vi "test_char limit case 1.vi"(8 "error in (no error)":errorcluster, 11 "TestCase in":refnum<class "Char Count Limit.lvclass">) -> (0 "error out":errorcluster, 3 "TestCase out":refnum<class "Char Count Limit.lvclass">)   [LabVIEW 2017, in "Char Count Limit.lvclass"]
uses:
  Char Count Limit.lvclass
  <vilib>/addons/_JKI Toolkits/VI Tester/TestCase.llb/TestCase.lvclass
  Libraries/SSH/SSH.lvlib
  C:/Program Files (x86)/National Instruments/LabVIEW 2017/vi.lib/addons/_JKI Toolkits/VI Tester/TestCase.llb/TestCase.lvclass
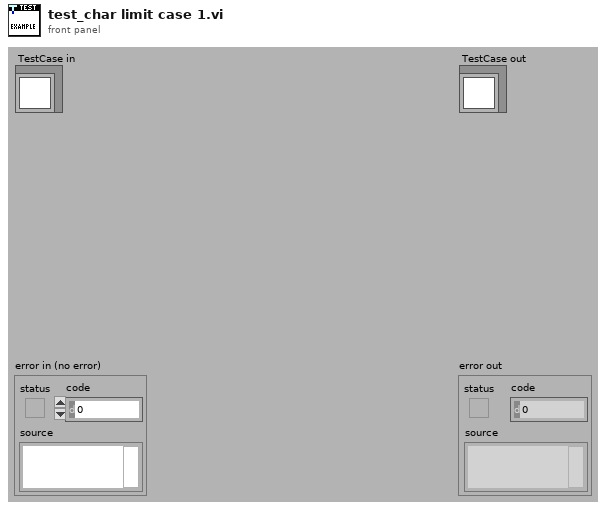
[diagram p1: front panel]
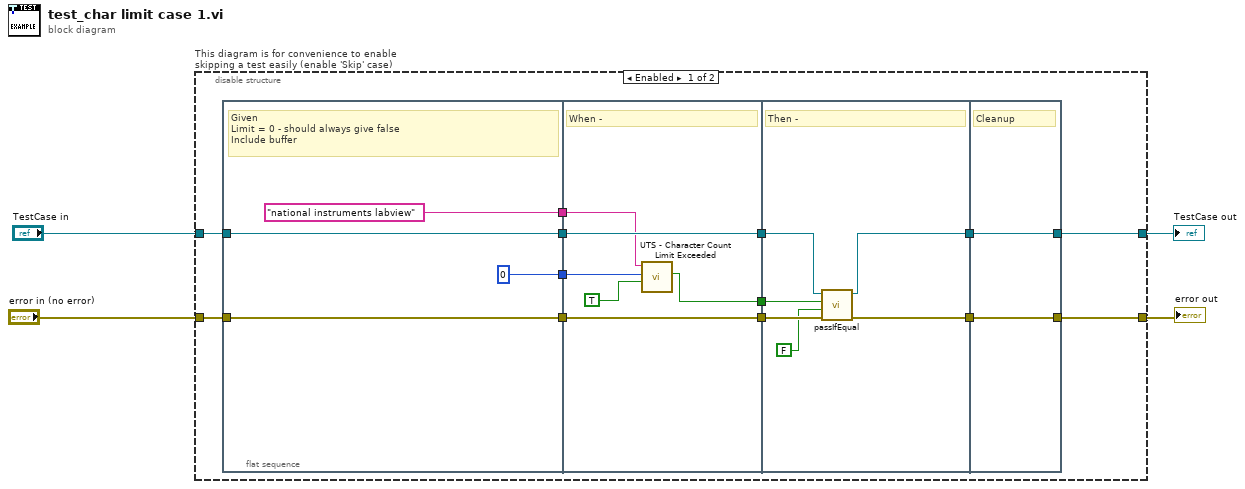
[diagram p0: block diagram]
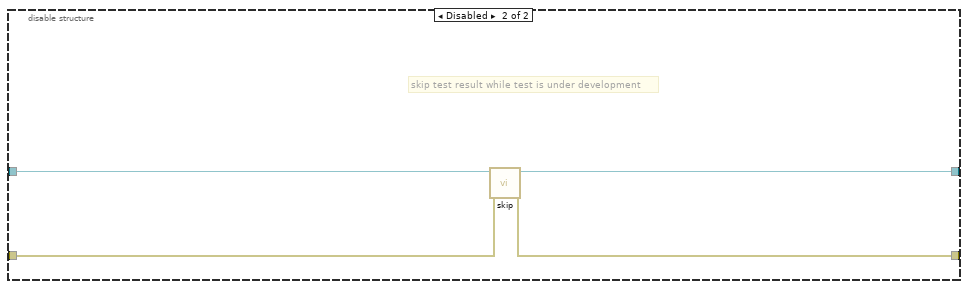
[diagram p2: hidden frame]
diagram:
  n1 = disable-structure "This diagram is for convenience to enable skipping a test easily (enable 'Skip' case)" shown="Enabled" {
    disable-tunnel: "TestCase in" -> [w11 w39]
    disable-tunnel: [w9 w37] -> w1
    disable-tunnel: [w8 w38] -> w3
    disable-tunnel: "error in (no error)" -> [w10 w36]
    frame Enabled {
      n2 = flat-sequence {
        tunnel: w10 -> [w20]
        tunnel: w11 -> [w21]
        tunnel: [w21] -> w17
        tunnel: [w20] -> w16
        tunnel: ["national instruments labview" ("Response String in")] -> w7
        tunnel: [0 ("Character Count Limit")] -> w6
        tunnel: [w27] -> w15
        tunnel: [w26] -> w14
        tunnel: w17 -> [w27]
        tunnel: w16 -> [w26]
        tunnel: w7 -> [w25]
        tunnel: w6 -> [w24]
        tunnel: [w23] -> w5
        tunnel: [w32] -> w13
        tunnel: [w30] -> w12
        tunnel: w15 -> [w33]
        tunnel: w14 -> [w31]
        tunnel: w5 -> [w29]
        tunnel: [w34] -> w8
        tunnel: [w35] -> w9
        tunnel: w13 -> [w35]
        tunnel: w12 -> [w34]
        frame #0 {
          # "Given\nLimit = 0 - should always give false\nInclude buffer"
        }
        frame #1 {
          # "When -"
          n3 = call "UTS - Character Count Limit Exceeded.vi"("Include Buffer"=TRUE, "Character Count Limit"=w24, "Response String in"=w25) -> ("Limit Exceeded"=w23:bool)  [unwired: 8 in]
        }
        frame #2 {
          # "Then -"
          n4 = call-dynamic "passIfEqual.vi"("error in (no error)"=w31, "y"=FALSE, "x"=w29, "TestCase in"=w33) -> ("error out"=w30:errorcluster, "TestCase out"=w32:refnum<class "Char Count Limit.lvclass">)  [unwired: 6 in]
        }
        frame #3 {
          # "Cleanup"
        }
      }
    }
    frame Disabled {
      # "skip test result while test is under development"
      n5 = call <vilib>:"skip.vi"("error in (no error)"=w36, "TestCase in"=w39) -> ("error out"=w38:errorcluster, "TestCase out"=w37:refnum<class "Char Count Limit.lvclass">)  [unwired: 8 in]
    }
  }
  "error out" <- w3
  "TestCase out" <- w1
